vi "INIT CreateEngineChannels.vi"(8 "error in (no error)":errorcluster, 11 "Device Item Ref in":T1 format="%.0x") -> (0 "error out":errorcluster, 3 "Device Item Ref out":T1 format="%.0x")   [LabVIEW 2018, in "CAN Gateway System Explorer.lvlib"]
uses:
  CAN Gateway System Explorer.lvlib
  <vilib>/NI Veristand/Custom Device API/Custom Device Item Ref.ctl
  <vilib>/NI Veristand/Custom Device API/Custom Device Channel.ctl
  <vilib>/NI Veristand/Custom Device API/Custom Device Channel Type.ctl
  Shared/Constants.vi
  <vilib>/NI Veristand/Custom Device API/Custom Device API.lvlib
  Shared/CAN Gateway Shared.lvlib
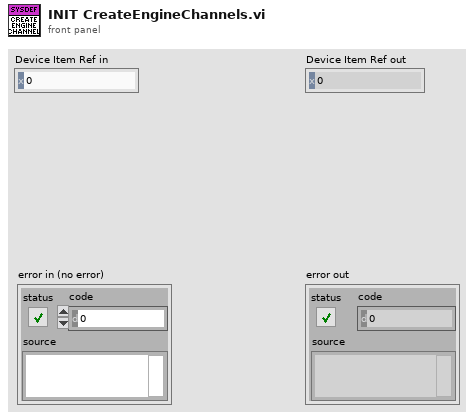
[diagram p1: front panel]
types:
  T1 = typedef "Custom Device API.lvlib/Custom Device Item Ref.ctl" = u64
  T2 = typedef "Custom Device API.lvlib/Custom Device Channel.ctl" = cluster{"Type":T3, "Units":string, "Default Value":dbl, "Faultable":bool, "Scalable":bool}
  T3 = typedef "Custom Device API.lvlib/Custom Device Channel Type.ctl" = enum16{"Input", "Output"}
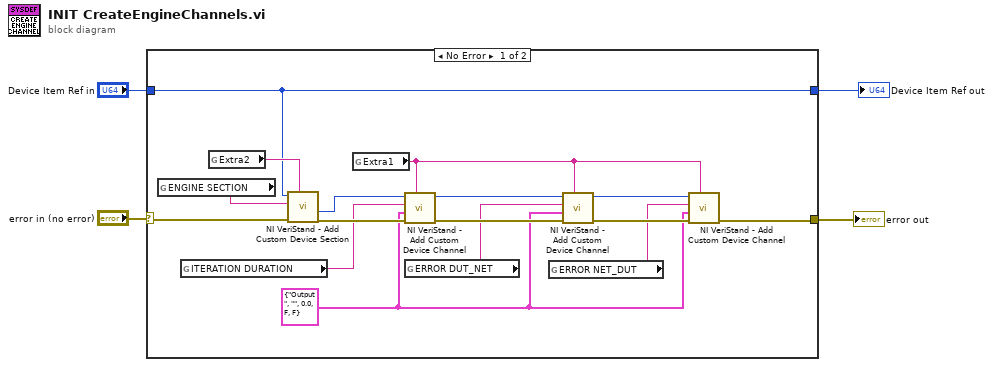
[diagram p0: block diagram]
diagram:
  n1 = case shown="No Error" "error in (no error)" {
    selector: "error in (no error)" -> [w20 w21]
    tunnel: "Device Item Ref in" -> [w5 w22]
    tunnel: [w14 w21] -> w2
    tunnel: [w5 w22] -> w1
    frame No Error {
      w11 = T2 {"Type"=enum."Output", "Units"="", "Default Value"=0.0, "Faultable"=FALSE, "Scalable"=FALSE} ("Channel")
      n2 = global read "Constants.vi" "ENGINE SECTION"() -> (w19:string)
      n3 = global read "Constants.vi" "ITERATION DURATION"() -> (w12:string)
      n4 = global read "Constants.vi" "Extra2"() -> (w18:string)
      n5 = call <vilib>:"NI VeriStand - Add Custom Device Section.vi"("GUID (Default Section)"=w18, "error in (no error)"=w20, "Section Name"=w19, "Parent Ref in"=w5) -> ("error out"=w17:errorcluster, "Section Ptr"=w13:T1)  [unwired: 4 in, 2 out]
      n6 = global read "Constants.vi" "Extra1"() -> (w6:string)
      n7 = call <vilib>:"NI VeriStand - Add Custom Device Channel.vi"("GUID (Default Channel)"=w6, "error in (no error)"=w17, "Channel"=w11, "Channel Name"=w12, "Parent Ref in"=w13) -> ("error out"=w16:errorcluster, "Parent Ref out"=w9:T1)  [unwired: 3 in, 2 out]
      n8 = global read "Constants.vi" "ERROR DUT_NET"() -> (w10:string)
      n9 = global read "Constants.vi" "ERROR NET_DUT"() -> (w8:string)
      n10 = call <vilib>:"NI VeriStand - Add Custom Device Channel.vi"("GUID (Default Channel)"=w6, "error in (no error)"=w16, "Channel"=w11, "Channel Name"=w10, "Parent Ref in"=w9) -> ("error out"=w15:errorcluster, "Parent Ref out"=w7:T1)  [unwired: 3 in, 2 out]
      n11 = call <vilib>:"NI VeriStand - Add Custom Device Channel.vi"("GUID (Default Channel)"=w6, "error in (no error)"=w15, "Channel"=w11, "Channel Name"=w8, "Parent Ref in"=w7) -> ("error out"=w14:errorcluster)  [unwired: 3 in, 3 out]
    }
    frame Error {
    }
  }
  "error out" <- w2
  "Device Item Ref out" <- w1
